vi "Querier.vi"() -> ()   [LabVIEW 2014, in "Generic Instrument.lvlib" / "Generic Instrument.lvclass"]
uses:
  Generic Instrument.lvclass
panel:
  in  "write buffer":string
  in  "VISA resource name":refnum<visa-resource-name>
  out "read buffer":string
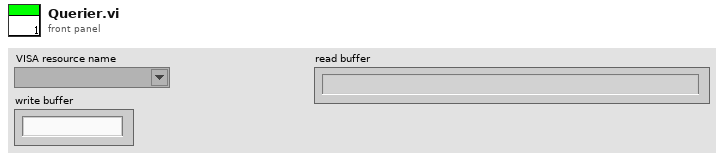
[diagram p1: front panel]
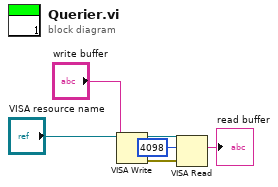
[diagram p0: block diagram]
diagram:
  n1 = VISA Write(VISA resource name="VISA resource name", write buffer="write buffer") -> (VISA resource name out=w6:refnum<visa-resource-name>, error out=w5:errorcluster)  [unwired: 1 in, 1 out]
  n2 = VISA Read(VISA resource name=w6, byte count=u32 4098, error in (no error)=w5) -> (read buffer=→"read buffer":string)  [unwired: 3 out]
